vi "Edit Data v2.vi"(2 "error in (no error)":errorcluster, 3 "History Data input":T2) -> (0 "error out":errorcluster, 1 "History Data output":T2)   [LabVIEW 2021]
doc: "Este VI se encarga de editar/recortar los datos de temperatura"
panel:
  in  "Quit":bool
  in  "Edit button":bool
  in  "Posicion final":dbl min=0.0 step=0.5
  in  "Posicion inicial":dbl min=0.0 step=0.5
  out "Temperature Data":T1(graph)=[{"Temp.Max"=27.3, "Temp.Actual"=25.6276741088368, "Temp.Min"=27.1}, {"Temp.Max"=27.3, "Temp.Actual"=25.73080566013232, "Temp.Min"=27.1}, {"Temp.Max"=27.3, "Temp.Actual"=25.74369710404426, "Temp.Min"=27.1}, {"Temp.Max"=27.3, "Temp.Actual"=25.74369710404426, "Temp.Min"=27.1}, {"Temp.Max"=27.3, "Temp.Actual"=25.74369710404426, "Temp.Min"=27.1}, {"Temp.Max"=27.3, "Temp.Actual"=25.74369710404426, "Temp.Min"=27.1}, {"Temp.Max"=27.3, "Temp.Actual"=25.846828655339777, "Temp.Min"=27.3}, {"Temp.Max"=27.3, "Temp.Actual"=25.885502987075597, "Temp.Min"=27.3}, {"Temp.Max"=27.3, "Temp.Actual"=25.898394430987537, "Temp.Min"=27.3}, {"Temp.Max"=27.3, "Temp.Actual"=25.898394430987537, "Temp.Min"=27.3}, {"Temp.Max"=30.3, "Temp.Actual"=25.937068762723356, "Temp.Min"=27.3}, {"Temp.Max"=30.3, "Temp.Actual"=26.001525982283056, "Temp.Min"=27.3}, {"Temp.Max"=30.3, "Temp.Actual"=26.014417426194996, "Temp.Min"=27.3}, {"Temp.Max"=30.3, "Temp.Actual"=26.040200314018875, "Temp.Min"=27.3}, {"Temp.Max"=27.3, "Temp.Actual"=26.065983201842755, "Temp.Min"=27.3}, {"Temp.Max"=27.3, "Temp.Actual"=26.130440421402454, "Temp.Min"=27.3}, {"Temp.Max"=27.3, "Temp.Actual"=26.156223309226334, "Temp.Min"=27.3}, {"Temp.Max"=27.3, "Temp.Actual"=26.182006197050214, "Temp.Min"=27.3}, {"Temp.Max"=27.3, "Temp.Actual"=26.233571972697973, "Temp.Min"=26.3}, {"Temp.Max"=27.3, "Temp.Actual"=26.285137748345733, "Temp.Min"=25.3}, {"Temp.Max"=27.3, "Temp.Actual"=26.272246304433793, "Temp.Min"=25.3}, {"Temp.Max"=27.3, "Temp.Actual"=26.272246304433793, "Temp.Min"=25.3}, {"Temp.Max"=27.3, "Temp.Actual"=26.336703523993492, "Temp.Min"=25.3}, {"Temp.Max"=30.3, "Temp.Actual"=26.362486411817372, "Temp.Min"=25.3}, {"Temp.Max"=30.3, "Temp.Actual"=26.41405218746513, "Temp.Min"=25.3}, {"Temp.Max"=30.3, "Temp.Actual"=26.43983507528901, "Temp.Min"=25.3}, {"Temp.Max"=30.3, "Temp.Actual"=26.46561796311289, "Temp.Min"=25.3}]
  # "Elige con que tramo quedarte y toma pasos múltiplos de 0,5"
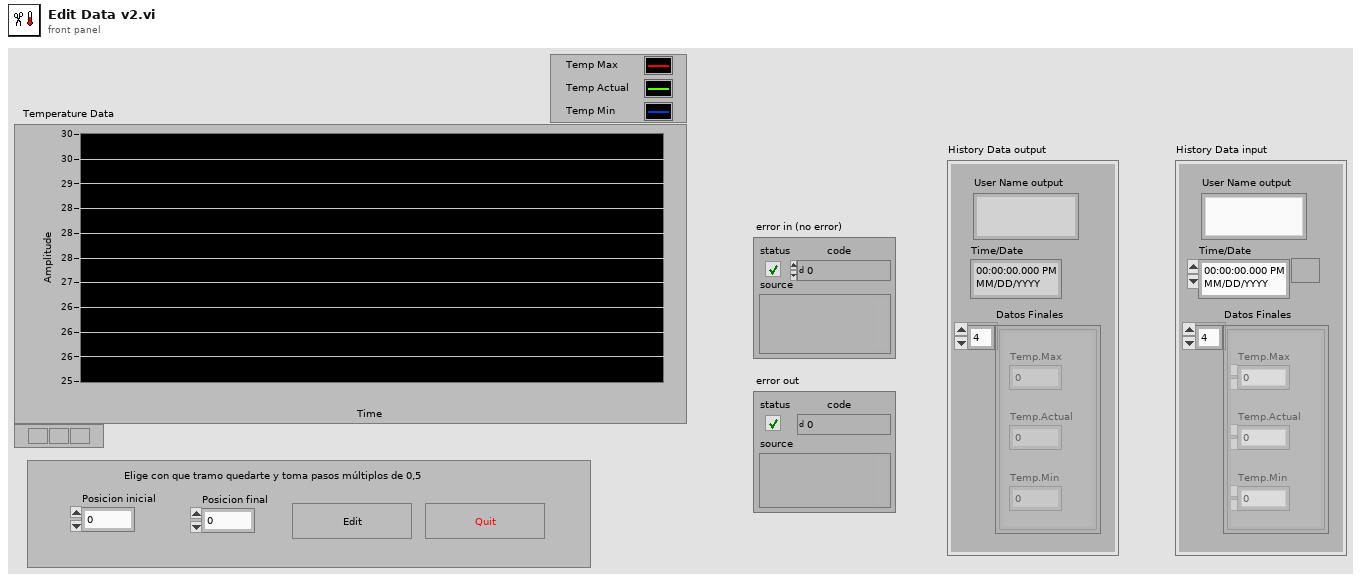
[diagram p1: front panel]
types:
  T1 = cluster{"Temp.Max":dbl, "Temp.Actual":dbl, "Temp.Min":dbl}[]
  T2 = cluster{"User Name output":string, "Time/Date":timestamp, "Datos Finales":cluster{"Temp.Max":dbl, "Temp.Actual":dbl, "Temp.Min":dbl}[]}
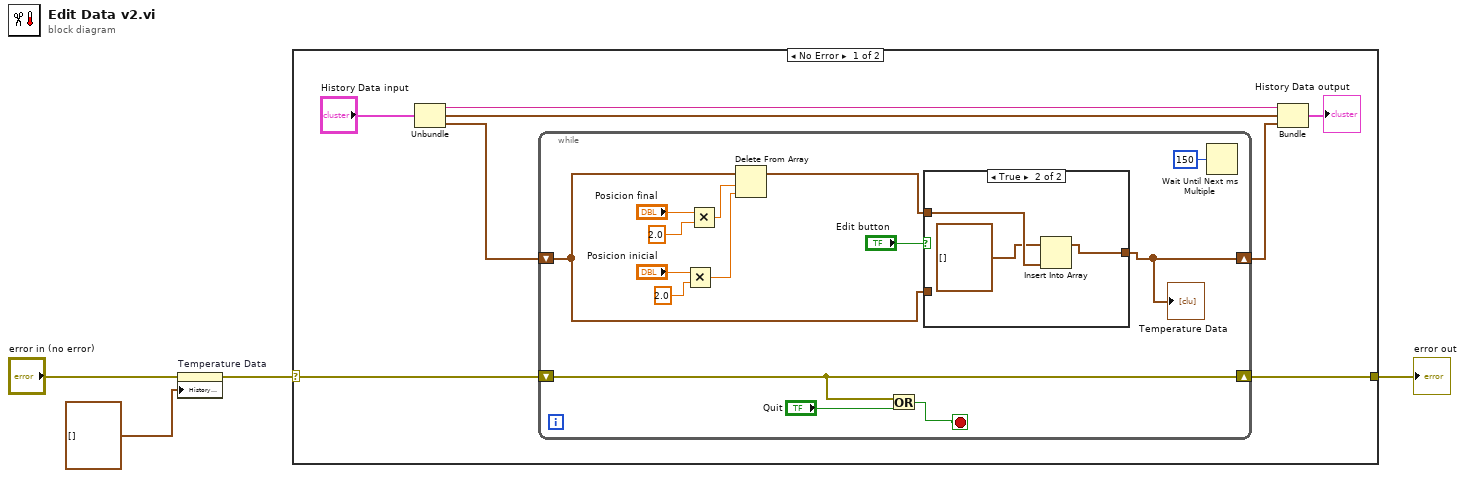
[diagram p0: block diagram]
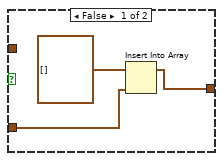
[diagram p2: hidden frame]
diagram:
  n1 = property on="Temperature Data" class="WFChart (strict)"(error in="error in (no error)", "History Data"=T1 []) -> (error out=w1:errorcluster)  [unwired: 1 in, 1 out]
  n2 = case shown="No Error" w1 {
    selector: w1 -> [w9 w33]
    tunnel: [w7 w33] -> w4
    frame No Error {
      n3 = Unbundle("History Data input") -> ("User Name output"=w11:string, "Time/Date"=w12:timestamp, "Datos Finales"=w8:T1)
      n4 = while {
        shift-right: [w19] -> w7
        shift-left: w9 -> [w19]
        shift-right: [w13] -> w5
        shift-left: w8 -> [w17]
        stop <- w20 stop-if-true
        n5 = Multiply(x="Posicion inicial", y=2.0) -> (x*y=w23:dbl)
        n6 = Multiply(x="Posicion final", y=2.0) -> (x*y=w25:dbl)
        n7 = Delete From Array(array=w17, length=w25, index=w23) -> (array with subset deleted=w18:T1)  [unwired: 1 out]
        n8 = Or(x=w19, y="Quit") -> (x .or. y?=w20:bool)
        n9 = case shown="True" "Edit button" {
          tunnel: w18 -> [_ w32]
          tunnel: w17 -> [w29 _]
          tunnel: [w27 w30] -> w13
          frame False {
            n10 = Insert Into Array(array=T1 [], new element=w29) -> (w27:T1)  [unwired: 1 in]
          }
          frame True {
            n11 = Insert Into Array(array=T1 [], new element=w32) -> (w30:T1)  [unwired: 1 in]
          }
        }
        "Temperature Data" <- w13
        n12 = Wait Until Next ms Multiple(millisecond multiple=u32 150) -> ()  [unwired: 1 out]
      }
      n13 = Bundle("User Name output"=w11, "Time/Date"=w12, "Datos Finales"=w5) -> (→"History Data output":T2)  [unwired: 1 in]
    }
    frame Error {
    }
  }
  "error out" <- w4
